vi "Custom Test Template.vi"(3 "Error In":errorcluster, 4 "Solution VI":path, 5 "User VI":path) -> (0 "Error Out":errorcluster, 2 "Results":T1={"Id"="", "Score"={"Status"=enum."Passed", "cpu_time"=-1, "max_memory"=-1, "style_score"=-1, "score0"="", "score1"="", "score2"="", "score3"="", "score4"="", "score5"=""}})   [LabVIEW 2013, in "VIChallenge.lvlib"]
doc: "This VI is a template for a custom users test. The User VI control will provide the absolute path to the VI to test. The solution VI control will provide the absolute path to the solution VI. The Results indicator should be populated with the results from testing the user submitted VI."
uses:
  <vilib>/LabVIEW Hacker/VIChallenge/VIChallenge.lvlib
  <vilib>/LabVIEW Hacker/VIChallenge/Private/Grader/Type Defs/UTF Status.ctl
  <vilib>/LabVIEW Hacker/VIChallenge/Private/Type Defs/Database/Score.ctl
  <vilib>/LabVIEW Hacker/VIChallenge/Private/Grader/Type Defs/Grader Result.ctl
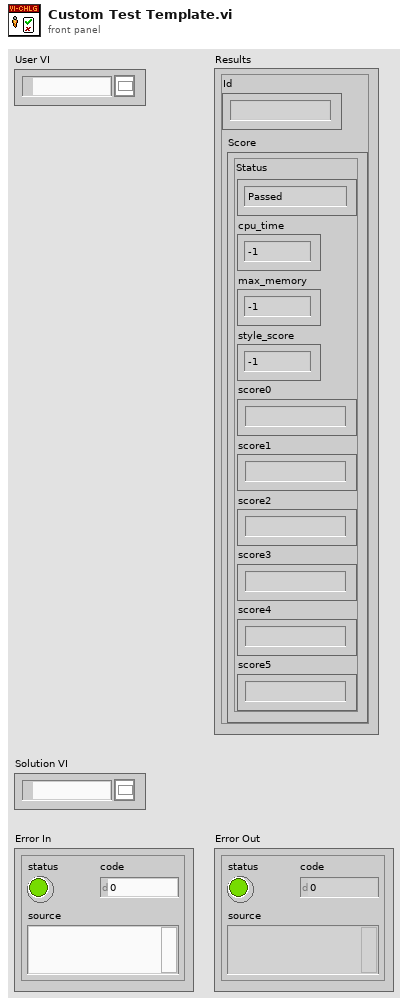
[diagram p1: front panel]
types:
  T1 = typedef "VIChallenge.lvlib/Grader Result.ctl" = cluster{"Id":string, "Score":T2}
  T2 = typedef "VIChallenge.lvlib/Score.ctl" = cluster{"Status":T3, "cpu_time":i32, "max_memory":i32, "style_score":i32, "score0":string, "score1":string, "score2":string, "score3":string, "score4":string, "score5":string}
  T3 = typedef "VIChallenge.lvlib/UTF Status.ctl" = enum16{"Null", "Passed", "Failed", "Error", "Skipped", "Not Processed"}
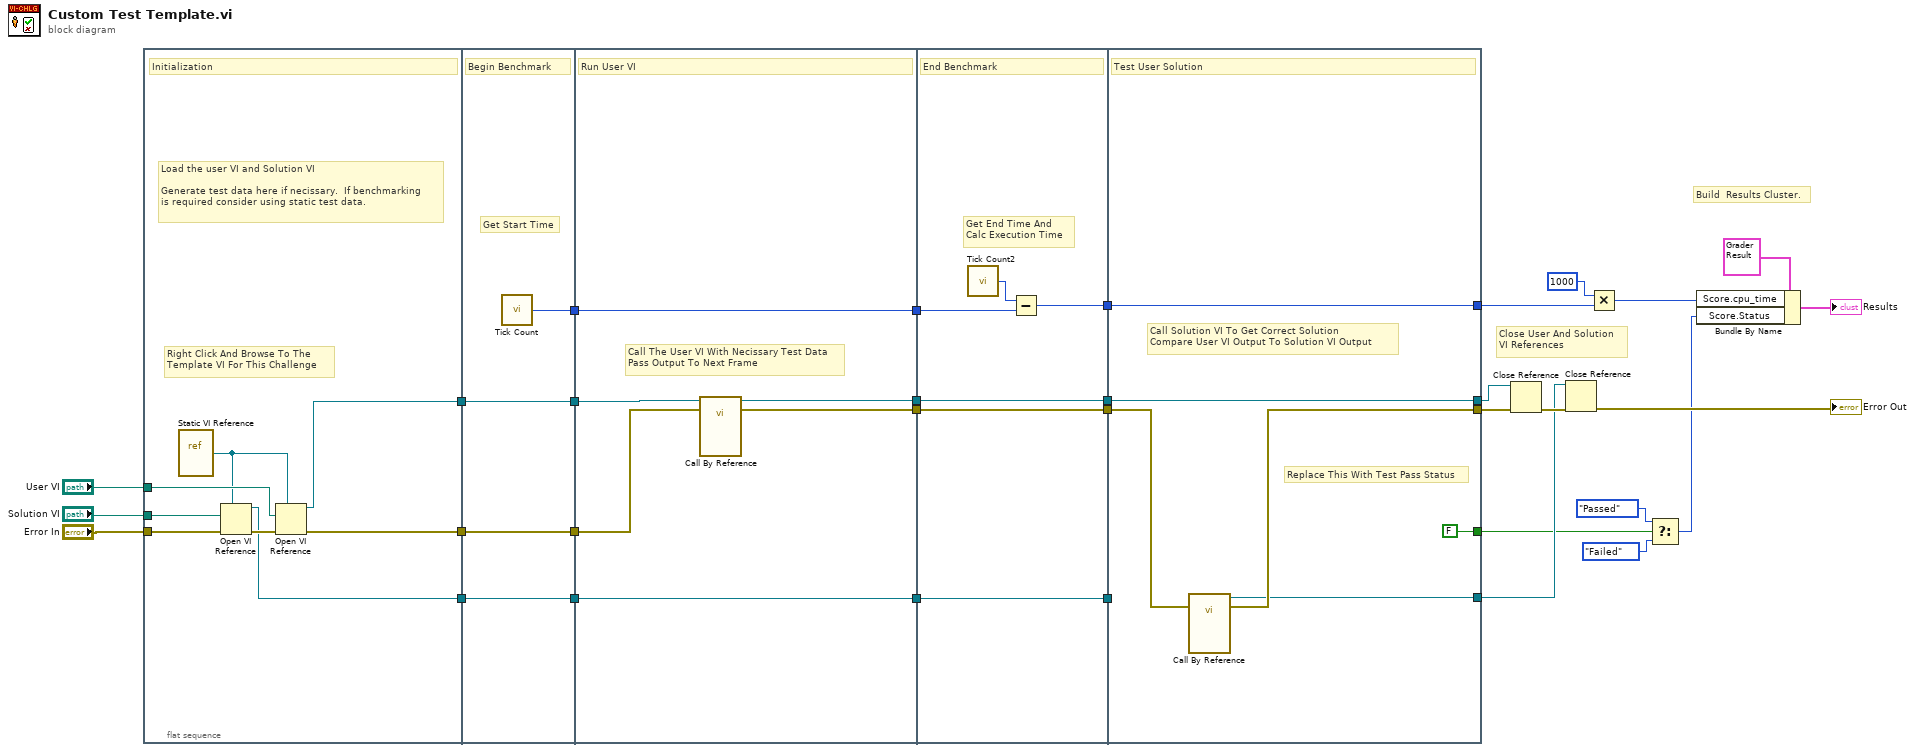
[diagram p0: block diagram]
diagram:
  # "Build  Results Cluster."
  # "Close User And Solution\nVI References"
  n1 = flat-sequence {
    tunnel: "User VI" -> [w40]
    tunnel: "Solution VI" -> [w39]
    tunnel: "Error In" -> [w37]
    tunnel: [w35] -> w29
    tunnel: [w34] -> w26
    tunnel: [w33] -> w24
    tunnel: w29 -> [w44]
    tunnel: [w44] -> w28
    tunnel: [w43] -> w27
    tunnel: w26 -> [w43]
    tunnel: [w42] -> w25
    tunnel: w24 -> [w42]
    tunnel: [w41] -> w21
    tunnel: w28 -> [w50]
    tunnel: w27 -> [w45]
    tunnel: w25 -> [w47]
    tunnel: [w49] -> w23
    tunnel: [w48] -> w22
    tunnel: w21 -> [w48]
    tunnel: [w47] -> w20
    tunnel: [w46] -> w17
    tunnel: w23 -> [w56]
    tunnel: w22 -> [w54]
    tunnel: w20 -> [w52]
    tunnel: [w56] -> w19
    tunnel: [w53] -> w18
    tunnel: w17 -> [w53]
    tunnel: [w52] -> w16
    tunnel: [w51] -> w2
    tunnel: w19 -> [w62]
    tunnel: [w61] -> w14
    tunnel: w18 -> [w60]
    tunnel: w16 -> [_]
    tunnel: [w60] -> w15
    tunnel: [w59] -> w12
    tunnel: [FALSE] -> w4
    tunnel: [w57] -> w3
    tunnel: w2 -> [w57]
    frame #0 {
      # "Load the user VI and Solution VI\n\nGenerate test data here if necissary.  If benchmarking \nis required consider using static test data."
      # "Right Click And Browse To The \nTemplate VI For This Challenge"
      # "Initialization"
      n2 = vi-ref "Static VI Reference"() -> ("vi reference"=w38:refnum<vi>)
      n3 = Open VI Reference(type specifier VI Refnum (for type only)=w38, vi path=w39, error in (no error)=w37) -> (vi reference=w33:refnum<vi>, error out=w36:errorcluster)  [unwired: 3 in]
      n4 = Open VI Reference(type specifier VI Refnum (for type only)=w38, vi path=w40, error in (no error)=w36) -> (vi reference=w34:refnum<vi>, error out=w35:errorcluster)  [unwired: 3 in]
    }
    frame #1 {
      # "Get Start Time"
      # "Begin Benchmark"
      n5 = call "Tick Count"() -> ("Tick Count(uSec)"=w41:u32)
    }
    frame #2 {
      # "Call The User VI With Necissary Test Data\nPass Output To Next Frame"
      # "Run User VI"
      n6 = call-by-ref "?"(reference=w45, error in=w50) -> (reference out=w46:refnum<vi>, error out=w49:errorcluster)
    }
    frame #3 {
      # "Get End Time And \nCalc Execution Time"
      # "End Benchmark"
      n7 = call "Tick Count2"() -> ("Tick Count(uSec)"=w55:u32)
      n8 = Subtract(x=w55, y=w54) -> (x-y=w51:u32)
    }
    frame #4 {
      # "Replace This With Test Pass Status"
      # "Call Solution VI To Get Correct Solution\nCompare User VI Output To Solution VI Output"
      # "Test User Solution"
      n9 = call-by-ref "?"(error in=w62) -> (reference out=w59:refnum<vi>, error out=w61:errorcluster)  [unwired: 1 in]
    }
  }
  n10 = Close Reference(reference=w15, error in (no error)=w14) -> (error out=w13:errorcluster)
  n11 = Close Reference(reference=w12, error in (no error)=w13) -> (error out=→"Error Out":errorcluster)
  n12 = Multiply(x=u32 1000 ("y"), y=w3) -> (x*y=w1:u32)
  n13 = Select(t=UTF_Status."Passed" ("Score.Status"), s=w4, f=UTF_Status."Failed" ("Score.Status")) -> (s? t:f=w5:T3)
  n14 = Bundle By Name(cluster=T1 {"Id"="", "Score"={"Status"=enum."Passed", "cpu_time"=-1, "max_memory"=-1, "style_score"=-1, "score0"="", "score1"="", "score2"="", "score3"="", "score4"="", "score5"=""}} ("Results"), "Score.cpu_time"=w1, "Score.Status"=w5) -> (→"Results":T1)
